vi "dataUnpackError.vi"(8 "errorIn":errorcluster, 11 "data":variant) -> (0 "errorOut":errorcluster, 3 "error":errorcluster)   [LabVIEW 2017]
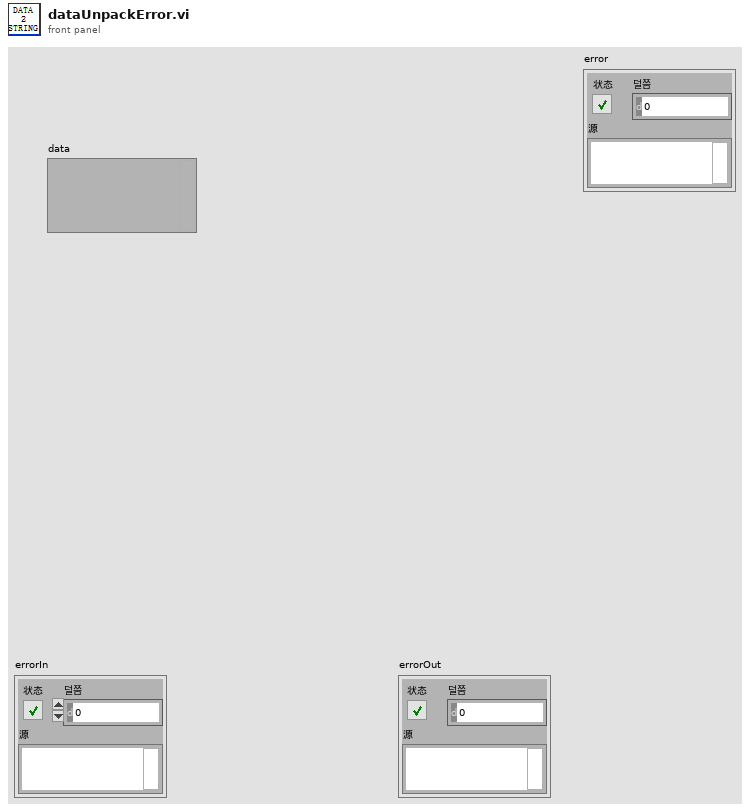
[diagram p1: front panel]
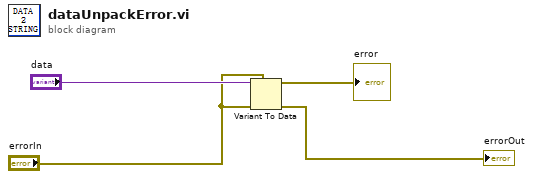
[diagram p0: block diagram]
diagram:
  n1 = Variant To Data(error in="errorIn", type="errorIn", Variant="data") -> (data=→"error":errorcluster, error out=→"errorOut":errorcluster)
